vi "acq.Single.Save.vi"(7 "DVR":T1, 8 "error in":errorcluster, 11 "buffer in":u16[][](array[numeric])) -> (0 "error out":errorcluster)   [LabVIEW 2020]
uses:
  _controls/data.ctl
  camera/camera.lvclass
  _controls/data.ref.ctl
  <vilib>/vision/Image Controls.llb/IMAQ Image.ctl
  _controls/state.ctl
  _controls/data.vars.ctl
  _controls/save_options.ctl
  _controls/flip.ctl
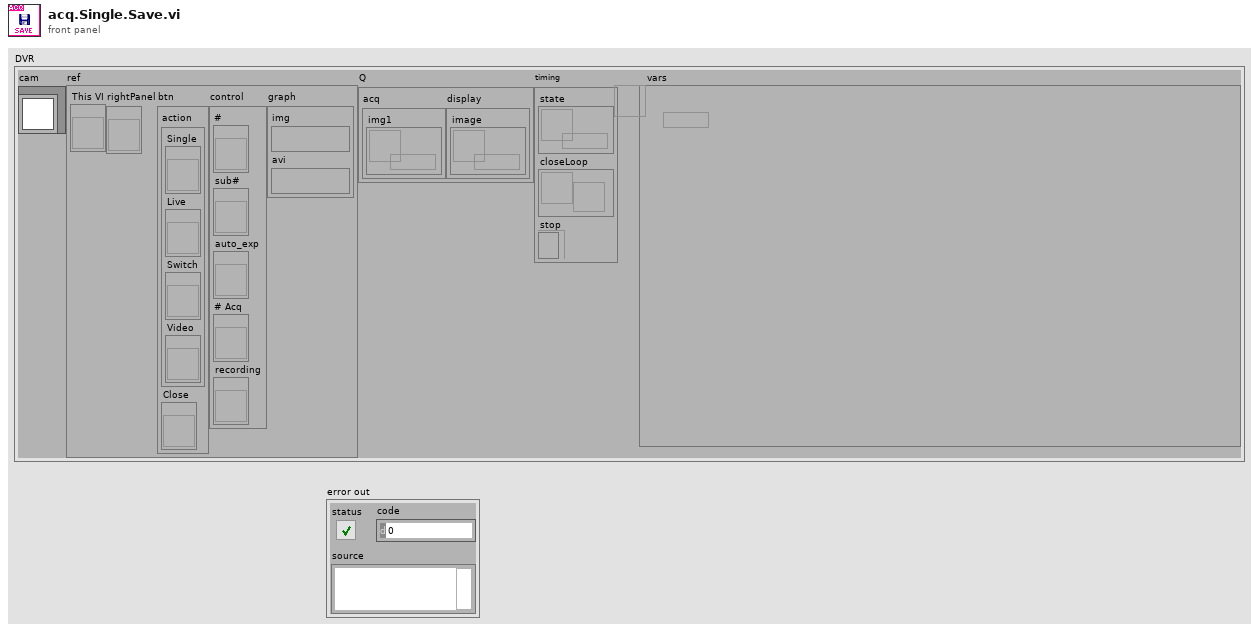
[diagram p1: front panel]
types:
  T1 = typedef "data.ctl" = cluster{"cam":refnum<class "camera.lvclass">, "ref":T2, "Q":cluster{"acq":cluster{"img1":refnum<queue>}, "display":cluster{"image":refnum<queue>}}, "timing":cluster{"state":refnum<queue>, "closeLoop":refnum<notifier>, "stop":refnum<k4>}, "vars":refnum<data-value>}
  T2 = typedef "data.ref.ctl" = cluster{"This VI":refnum<vi>, "rightPanel":refnum<vi>, "btn":cluster{"action":cluster{"Single":refnum<vi>, "Live":refnum<vi>, "Switch":refnum<vi>, "Video":refnum<vi>}, "Close":refnum<vi>}, "control":cluster{"#":refnum<vi>, "sub#":refnum<vi>, "auto_exp":refnum<vi>, "# Acq":refnum<vi>, "recording":refnum<vi>}, "graph":cluster{"img":T3, "avi":T3}}
  T3 = typedef "IMAQ Image.ctl" = refnum<image>
  T4 = typedef "data.vars.ctl" = cluster{"save":cluster{"base_folder":cluster{"Folder":path, "tif":bool, "jpg":bool}, "module":string, "#":u32, "sub#":u8, "save.op":T5, "same?":bool, "Shift":enum16{"Single", "Leapfrog"}, "jpg?":bool, "flip":T6}, "acq":cluster{"# Acq":u16, "rotate":bool, "FPS":dbl}, "calib.manual":cluster{"BG":cluster{"Image":u16[][], "enabled?":bool}, "FF":cluster{"Image":u16[][], "enabled?":bool}}}
  T5 = typedef "save_options.ctl" = enum16{"Light", "Full"}
  T6 = typedef "flip.ctl" = cluster{"x":bool, "y":bool}
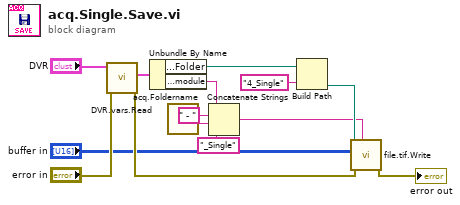
[diagram p0: block diagram]
diagram:
  n1 = call "DVR.vars.Read.vi"("error in"="error in", "DVR.state"="DVR") -> ("error out"=w4:errorcluster, "vars"=w12:T4)  [unwired: 8 in]
  n2 = Unbundle By Name(w12) -> ("save.base_folder.Folder"=w7:path, "save.module"=w14:string)
  n3 = call "acq.Foldername.vi"() -> ("foldernme"=w11:string)  [unwired: 11 in]
  n4 = Concatenate Strings(w14, " - " ("string"), w11, "_Single" ("string")) -> (w6:string)
  n5 = Build Path(base path=w7, name or relative path="4_Single" ("string")) -> (appended path=w10:path)
  n6 = call "file.tif.Write.vi"("name"=w6, "error in"=w4, "u16 pixmap"="buffer in", "path"=w10) -> ("error out"=→"error out":errorcluster)  [unwired: 7 in]
